vi "CSDB_Common.Listbox.size to text.vi"(1 "listbox ref":refnum<vi>) -> ()   [LabVIEW 2014, in "CSDB_Common.lvlib"]
uses:
  CSDB_Common.lvlib
panel:
  in  "Numeric":dbl caption="SuperProc"
  in  "dummy Listbox":i32[](listbox)
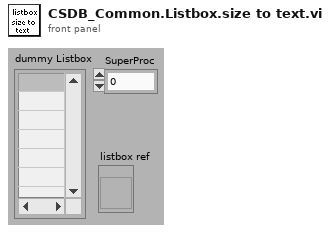
[diagram p1: front panel]
types:
  T1 = typedef "LVRowAndColumnTypeDef.ctl" = cluster{"Row":i32, "Column":i32}
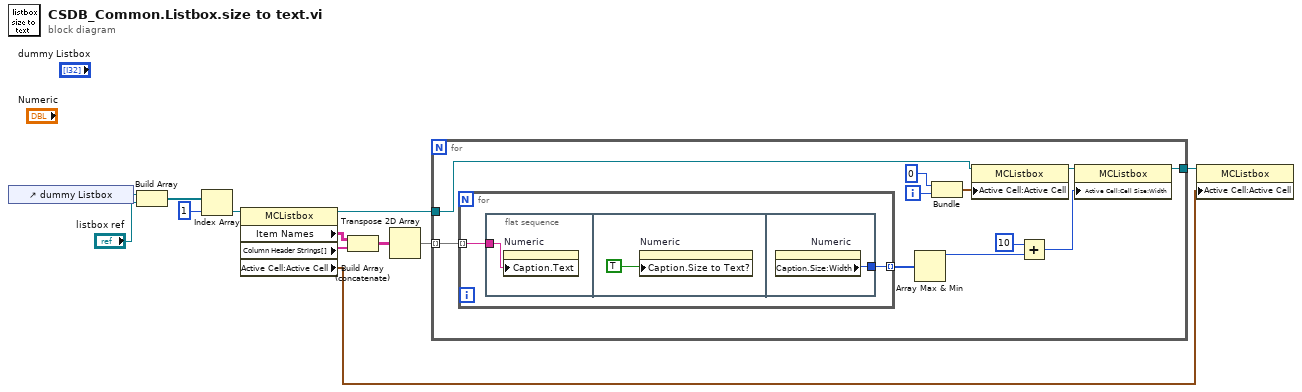
[diagram p0: block diagram]
diagram:
  n1 = control-ref of="dummy Listbox"() -> (w12:refnum<vi>)
  n2 = Build Array(w12, "listbox ref") -> (w10:refnum<vi>[])
  n3 = Index Array(array=w10, index=1) -> (element=w8:refnum<vi>)
  n4 = property class="MCListbox"(reference=w8) -> (reference out=w6:refnum<vi>, "Item Names"=w3:string[][], "Column Header Strings[]"=w2:string[], "Active Cell:Active Cell"=w4:T1)  [unwired: 1 in, 1 out]
  n5 = Build Array (concatenate)(w3, w2) -> (w1:string[][])
  n6 = Transpose 2D Array(2D array=w1) -> (transposed array=w7:string[][])
  n7 = for {
    tunnel: w7 -> [w23] mode=indexing
    tunnel: w6 -> [w17]
    tunnel: [w14] -> w5
    i -> [w13]
    n8 = for {
      tunnel: [w25] -> w20 mode=indexing
      tunnel: w23 -> [w24] mode=indexing
      n9 = flat-sequence {
        tunnel: w24 -> [w26]
        tunnel: [w28] -> w25
        frame #0 {
          n10 = property on="Numeric" class="DigNum (strict)"("Caption.Text"=w26) -> ()  [unwired: 2 in, 2 out]
        }
        frame #1 {
          n11 = property on="Numeric" class="DigNum (strict)"("Caption.Size to Text?"=TRUE ("Caption.Size to Text")) -> ()  [unwired: 2 in, 2 out]
        }
        frame #2 {
          n12 = property on="Numeric" class="DigNum (strict)"() -> ("Caption.Size:Width"=w28:u32)  [unwired: 2 in, 2 out]
        }
      }
    }
    n13 = Array Max & Min(array=w20) -> (max value=w21:u32)  [unwired: 3 out]
    n14 = Bundle(0, w13) -> (w19:cluster{i32, i32})  [unwired: 1 in]
    n15 = property class="MCListbox"(reference=w17, "Active Cell:Active Cell"=w19) -> (reference out=w16:refnum<vi>)  [unwired: 1 in, 1 out]
    n16 = Add(x=u32 10, y=w21) -> (x+y=w15:u32)
    n17 = property class="MCListbox"(reference=w16, "Active Cell:Cell Size:Width"=w15) -> (reference out=w14:refnum<vi>)  [unwired: 1 in, 1 out]
  }
  n18 = property class="MCListbox"(reference=w5, "Active Cell:Active Cell"=w4) -> ()  [unwired: 1 in, 2 out]
